vi "PI_Image_Scanner_Prepare.vi"(0 "x-Pixel":u16=100, 1 "y-Pixel":u16=100, 3 "Picture size x":dbl=20.0 min=0.1 max=200.0 format="%1.1f um", 4 "Picture size y":dbl=20.0 min=0.1 max=200.0 format="%1.1f um", 7 "Axis":enum32{"x-y", "x-z", "y-z"}(ring), 9 "Scanner Divider":i32) -> (14 "Commandset out":string[](array[string]), 16 "Measurement time / [s]":i32)   [LabVIEW 2010]
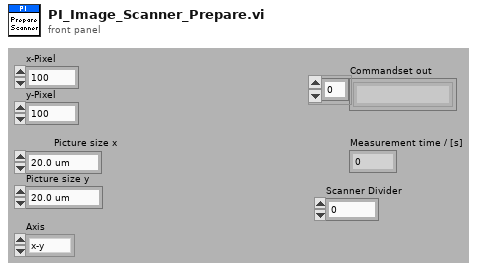
[diagram p1: front panel]
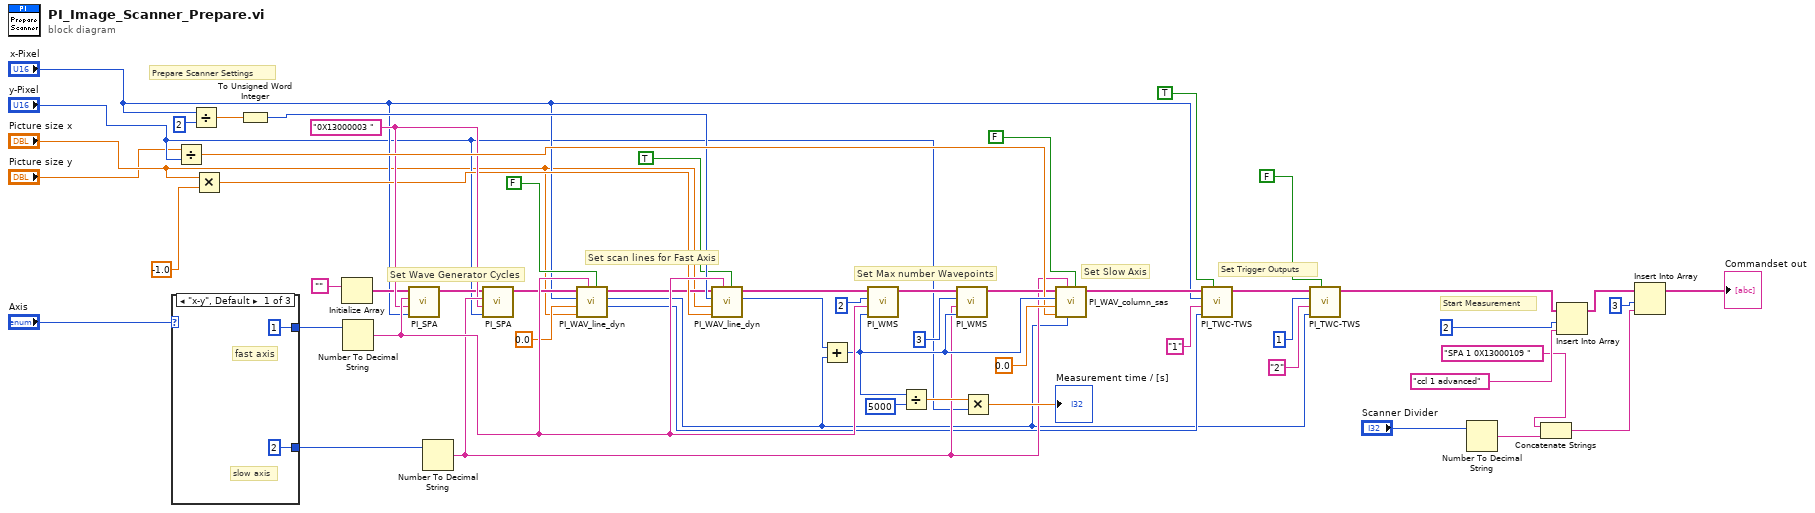
[diagram p0: block diagram]
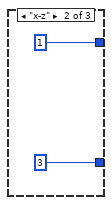
[diagram p2: hidden frame]
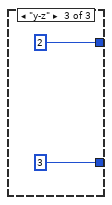
[diagram p3: hidden frame]
diagram:
  w40 = "0X13000003 " ("string")
  # "Start Measurement"
  # "Set Slow Axis"
  # "Set Trigger Outputs"
  # "Set Max number Wavepoints"
  # "Set scan lines for Fast Axis"
  # "Set Wave Generator Cycles"
  # "Prepare Scanner Settings"
  n1 = case shown="\"x-y\", Default" "Axis" {
    tunnel: [1 1 2] -> w26
    tunnel: [2 3 3] -> w27
    frame "x-y", Default {
      # "slow axis"
      # "fast axis"
    }
    frame "x-z" {
    }
    frame "y-z" {
    }
  }
  n2 = Divide(x="Picture size y", y="y-Pixel") -> (x/y=w48:dbl)
  n3 = Divide(x="x-Pixel", y=u16 2) -> (x/y=w32:dbl)
  n4 = Multiply(x="Picture size x", y=-1.0) -> (x*y=w34:dbl)
  n5 = To Unsigned Word Integer(number=w32) -> (unsigned 16bit integer=w33:u16)
  n6 = Initialize Array("") -> (w38:string[])  [unwired: 1 out]
  n7 = Number To Decimal String(number=w26) -> (decimal integer string=w55:string)  [unwired: 1 out]
  n8 = call "PI_SPA.vi"("Value"="x-Pixel", "Register"=w40, "Axis"=w55, "Commandset in"=w38) -> ("Commandset out"=w39:string[])  [unwired: 7 out]
  n9 = Number To Decimal String(number=w27) -> (decimal integer string=w46:string)  [unwired: 1 out]
  n10 = call "PI_SPA.vi"("Value"="y-Pixel", "Register"=w40, "Axis"=w46, "Commandset in"=w39) -> ("Commandset out"=w37:string[])  [unwired: 7 out]
  n11 = call "PI_WAV_line_dyn.vi"("Attach to wav"=FALSE, "Axis Identifier"=w55, "Amplitude / [mu]"="Picture size x", "Startpos / [mu]"=0.0, "Pixel per scan"="x-Pixel", "Commandset in"=w37) -> ("Curve-Start-Pixel"=w23:u16, "Num_Pix"=w16:u16, "Commandset out"=w29:string[])  [unwired: 3 out]
  n12 = call "PI_WAV_line_dyn.vi"("Attach to wav"=TRUE, "Axis Identifier"=w55, "Amplitude / [mu]"=w34, "Startpos / [mu]"="Picture size x", "Pixel per scan"=w33, "Commandset in"=w29) -> ("Num_Pix"=w36:u16, "Commandset out"=w41:string[])  [unwired: 4 out]
  n13 = Add(x=w36, y=w16) -> (x+y=w51:u16)
  n14 = call "PI_WMS.vi"("Pixels to reserve"=w51, "Axis"=w55, "Position / Commandset"=2, "Commandset in"=w41) -> ("Commandset out"=w42:string[])  [unwired: 7 out]
  n15 = Divide(x=w51, y=5000) -> (x/y=w53:dbl)
  n16 = call "PI_WMS.vi"("Pixels to reserve"=w51, "Axis"=w46, "Position / Commandset"=3, "Commandset in"=w42) -> ("Commandset out"=w47:string[])  [unwired: 7 out]
  n17 = Multiply(x=w53, y="y-Pixel") -> (x*y=→"Measurement time / [s]":dbl)
  n18 = call "PI_WAV_column_sas.vi"("Attach to wav"=FALSE, "Steps per Scan-line"=w16, "Axis Identifier"=w46, "Amplitude / [mu]"=w48, "Startpos / [mu]"=0.0, "Pixel per scan"=w51, "Commandset in"=w47) -> ("Commandset out"=w24:string[])  [unwired: 4 out]
  n19 = call "PI_TWC-TWS.vi"("TWC?"=TRUE, "Curve_Start_Pixel"=w23, "Axis Identifier"="1", "Pixel per scan"="x-Pixel", "Commandset in"=w24) -> ("Commandset out"=w20:string[])  [unwired: 6 out]
  n20 = call "PI_TWC-TWS.vi"("TWC?"=FALSE, "Curve_Start_Pixel"=w16, "Axis Identifier"="2", "Pixel per scan"=u16 1, "Commandset in"=w20) -> ("Commandset out"=w3:string[])  [unwired: 6 out]
  n21 = Number To Decimal String(number="Scanner Divider") -> (decimal integer string=w4:string)  [unwired: 1 in]
  n22 = Concatenate Strings("SPA 1 0X13000109 " ("Neues Element/Teil-Array"), w4) -> (w5:string)
  n23 = Insert Into Array(array=w3, index=2, new element="ccl 1 advanced" ("Neues Element/Teil-Array")) -> (w10:string[])
  n24 = Insert Into Array(array=w10, index=3, new element=w5) -> (→"Commandset out":string[])
